vi "Data_Bios.vi"(7 "error in (no error)":errorcluster) -> (0 "error out":errorcluster, 1 "Hora":string, 3 "Data":string)   [LabVIEW 2019]
panel:
  # "sync clock to NIST time"
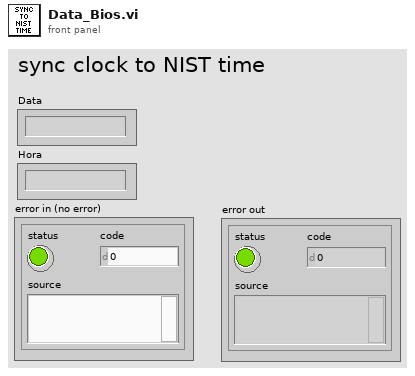
[diagram p1: front panel]
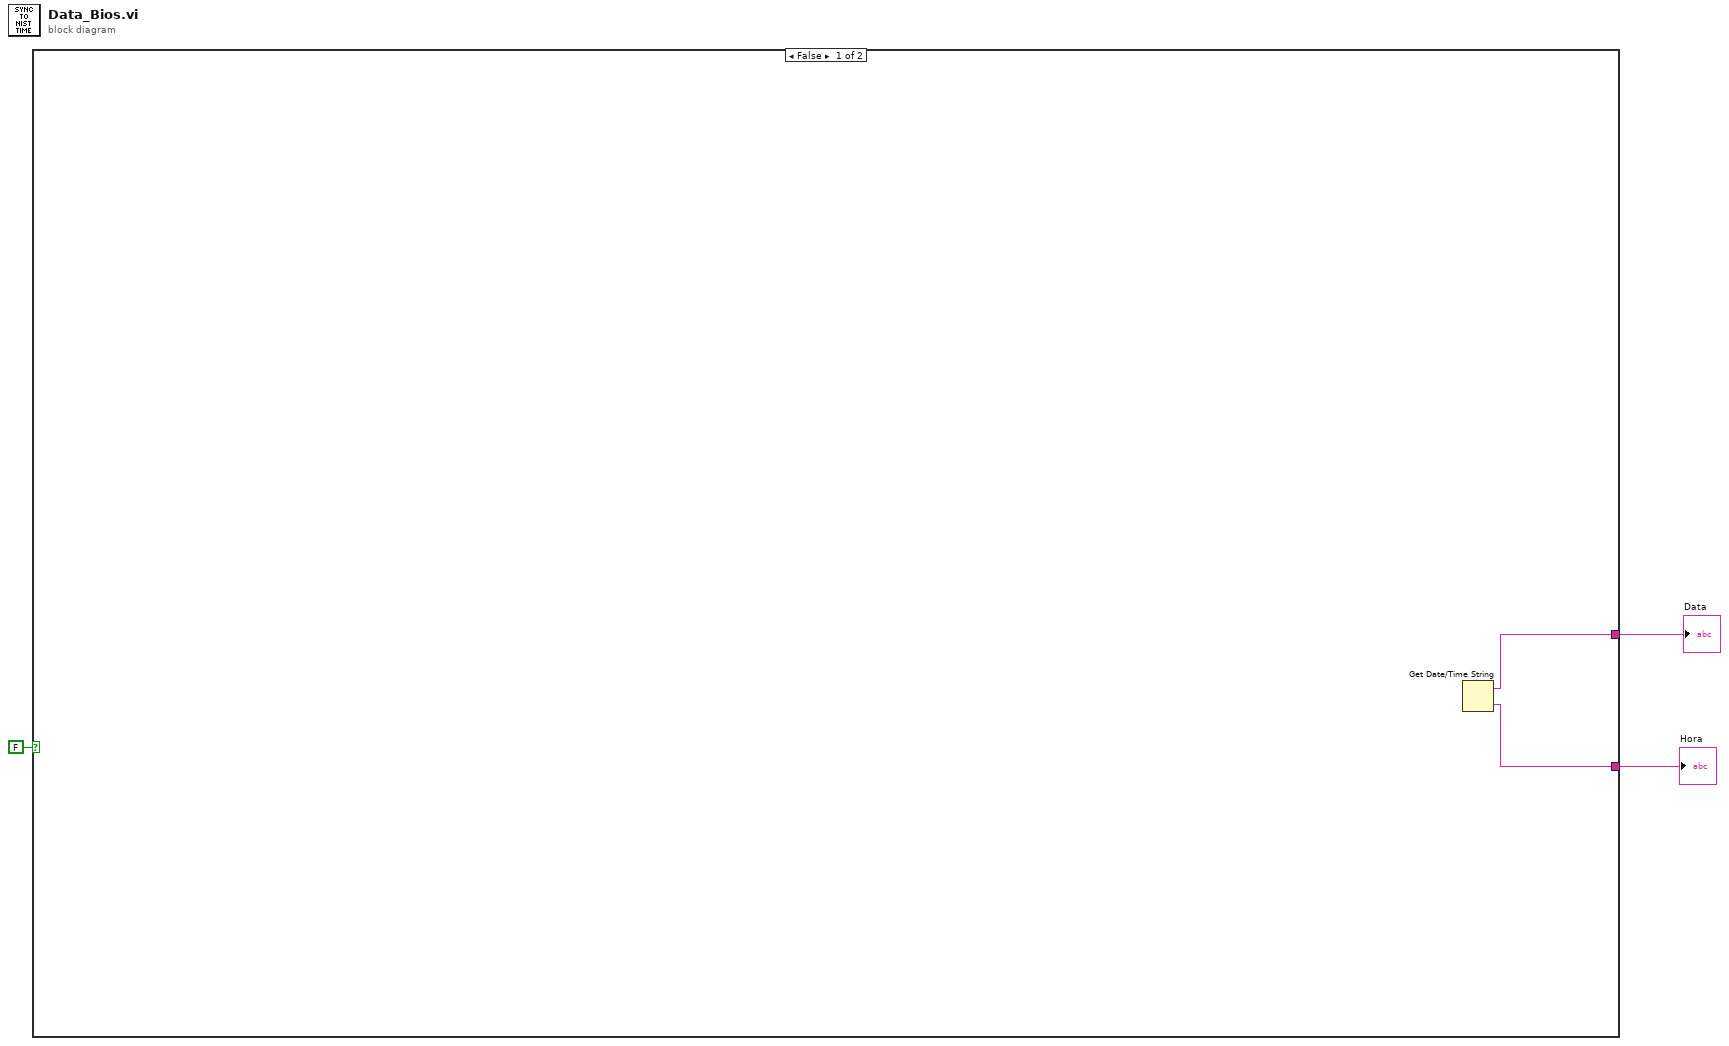
[diagram p0: block diagram]
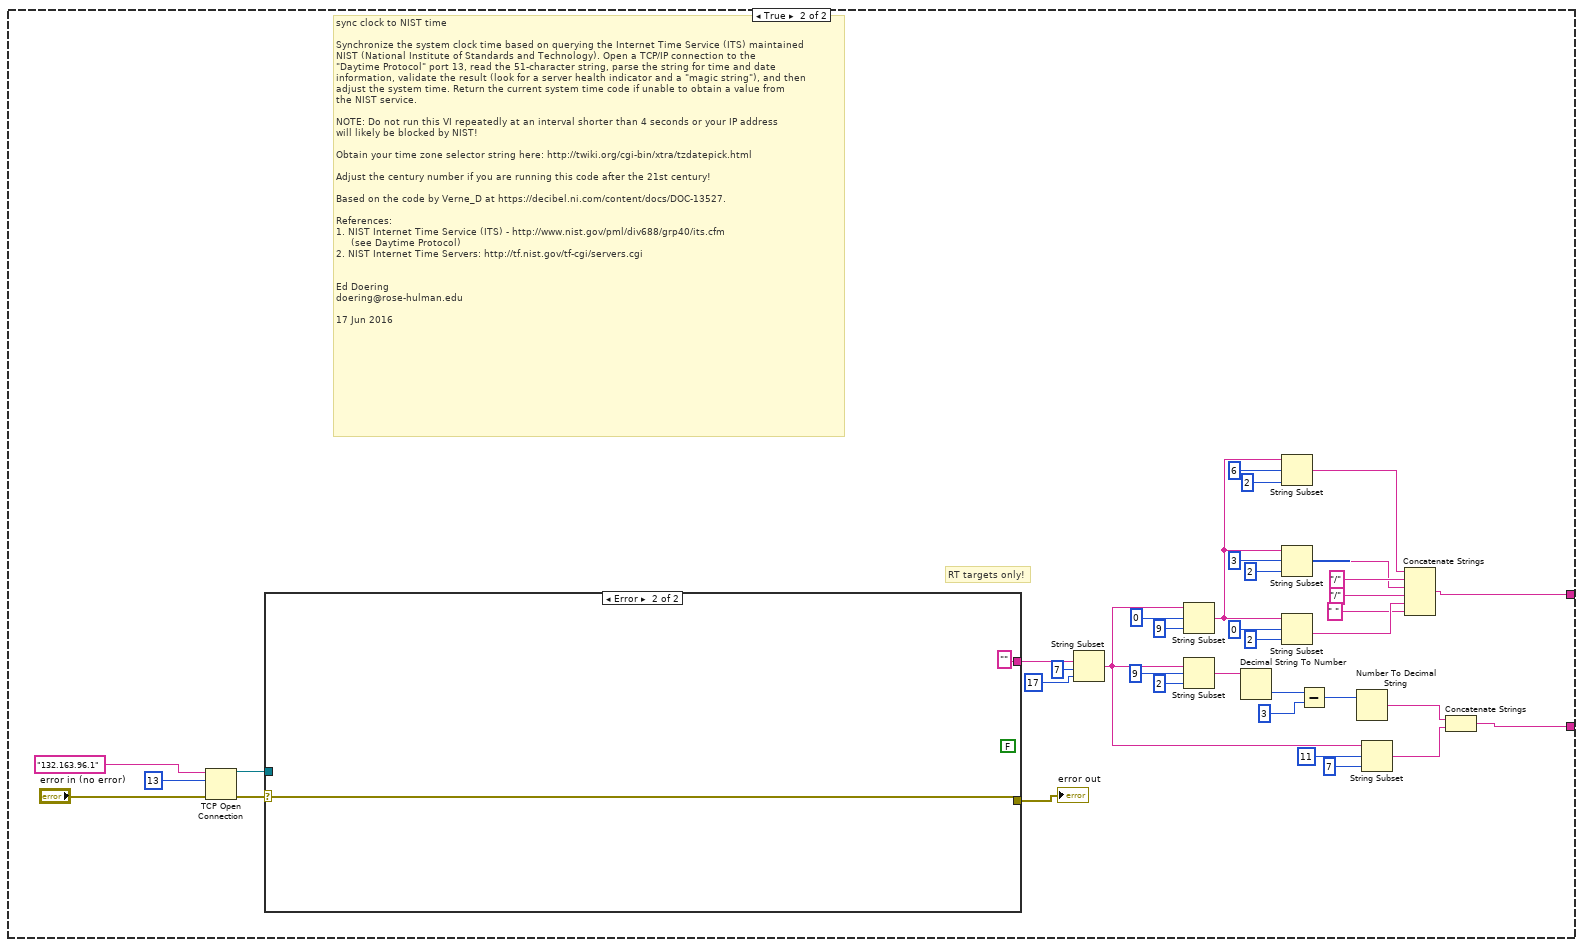
[diagram p2: hidden frame]
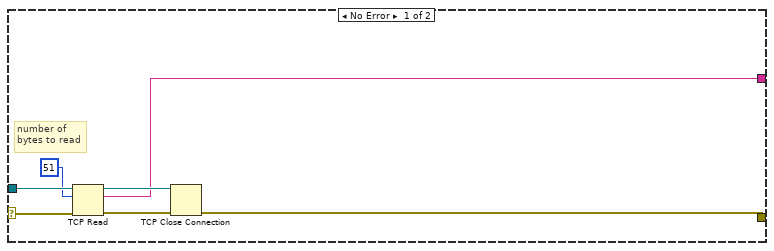
[diagram p3: hidden frame]
diagram:
  n1 = case shown="False" FALSE {
    tunnel: [w4 w7] -> w3
    tunnel: [w5 w6] -> w2
    frame False {
      n2 = Get Date/Time String() -> (date string=w5:string, time string=w4:string)  [unwired: 3 in]
    }
    frame True {
      # "RT targets only!"
      # "sync clock to NIST time\n\nSynchronize the system clock time based on querying the Internet Time Service (ITS) maintained\nNIST (National Institute of Standards and Technology). Open a TCP/IP connection to the\n\"Daytime Protocol\" port 13, read the 51-character string, parse the string for time and date \ninformation, validate the result (look for a server health indicator and a \"magic string\"), and then\nadjust the system time. Return the current system time code if unable to obtain a value from\nthe NIST service.\n\nNOTE: Do not run this VI repeatedly at an interval shorter than 4 seconds or your IP address\nwill likely be blocked by NIST!\n\nObtain your time zone selector string here: http://twiki.org/cgi-bin/xtra/tzdatepick.html \n\nAdjust the century number if you are running this code after the 21st century!\n\nBased on the code by Verne_D at https://decibel.ni.com/content/docs/DOC-13527.\n\nReferences:\n1. NIST Internet Time Service (ITS) - http://www.nist.gov/pml/div688/grp40/its.cfm\n     (see Daytime Protocol) \n2. NIST Internet Time Servers: http://tf.nist.gov/tf-cgi/servers.cgi \n\n\nEd Doering\ndoering@rose-hulman.edu\n\n17 Jun 2016"
      n3 = TCP Open Connection(address="132.163.96.1" ("NIST time server IP address"), remote port or service name=u16 13 ("port"), error in (no error)="error in (no error)") -> (connection ID=w39:refnum<k5>, error out=w40:errorcluster)  [unwired: 2 in]
      n4 = case shown="Error" w40 {
        selector: w40 -> [w49 w50]
        tunnel: w39 -> [w48 _]
        tunnel: [w43 w50] -> w38
        tunnel: [w45 "" ("data out")] -> w36
        frame No Error {
          # "number of\nbytes to read"
          n5 = TCP Read(connection ID=w48, bytes to read=51, error in (no error)=w49) -> (connection ID out=w46:refnum<k5>, data out=w45:string, error out=w47:errorcluster)  [unwired: 2 in]
          n6 = TCP Close Connection(connection ID=w46, error in (no error)=w47) -> (error out=w43:errorcluster)  [unwired: 1 in, 1 out]
        }
        frame Error {
          (unwired) FALSE
        }
      }
      "error out" <- w38
      n7 = String Subset(string=w36, offset (0)=7, length (rest)=17 ("length (rest)")) -> (substring=w26:string)
      n8 = String Subset(string=w26, offset (0)=0, length (rest)=9 ("length (rest)")) -> (substring=w19:string)
      n9 = String Subset(string=w26, offset (0)=9, length (rest)=2 ("length (rest)")) -> (substring=w32:string)
      n10 = Decimal String To Number(string=w32) -> (number=w31:i32)  [unwired: 2 in, 1 out]
      n11 = String Subset(string=w19, offset (0)=6, length (rest)=2 ("length (rest)")) -> (substring=w16:string)
      n12 = String Subset(string=w19, offset (0)=3, length (rest)=2 ("length (rest)")) -> (substring=w14:string)
      n13 = String Subset(string=w19, offset (0)=0, length (rest)=2 ("length (rest)")) -> (substring=w12:string)
      n14 = Subtract(x=w31, y=3) -> (x-y=w27:i32)
      n15 = Number To Decimal String(number=w27) -> (decimal integer string=w8:string)  [unwired: 1 in]
      n16 = String Subset(string=w26, offset (0)=11, length (rest)=7 ("length (rest)")) -> (substring=w9:string)
      n17 = Concatenate Strings(w16, "/" ("string"), w14, "/" ("string"), w12, " " ("string")) -> (w6:string)
      n18 = Concatenate Strings(w8, w9) -> (w7:string)
    }
  }
  "Data" <- w2
  "Hora" <- w3
